vi "read serial data.vi"(8 "error in (no error)":errorcluster, 11 "serial port":refnum<visa-resource-name>) -> (0 "error out":errorcluster, 1 "readings":T2[](array[typedef]), 2 "re-synch":bool, 3 "serial port out":refnum<visa-resource-name>)   [LabVIEW 2017]
uses:
  typedefs/reading.ctl
  typedefs/readingType.ctl
  typedefs/bytes in a reading.ctl
panel:
  out "bytes at port on fail":T1=20
  out "bytes read on fail":i32
  out "Serial Settings:Number of Bytes at Serial Port":u32
  out "wrong length":bool
  out "xsum fail":bool
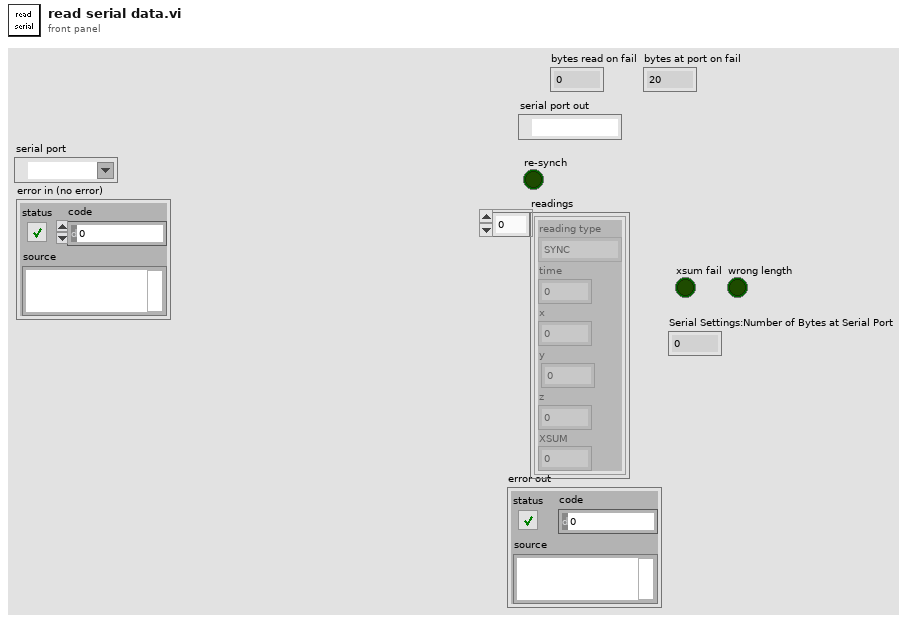
[diagram p1: front panel]
types:
  T1 = typedef "bytes in a reading.ctl" = u32
  T2 = typedef "reading.ctl" = cluster{"reading type":T3, "time":fxp<+,48,48>, "x":sgl, "y":sgl, "z":sgl, "XSUM":u8}
  T3 = typedef "readingType.ctl" = enum8{"SYNC", "DETVAL", "COILI", "MAGVEC", "ACCVEC"}
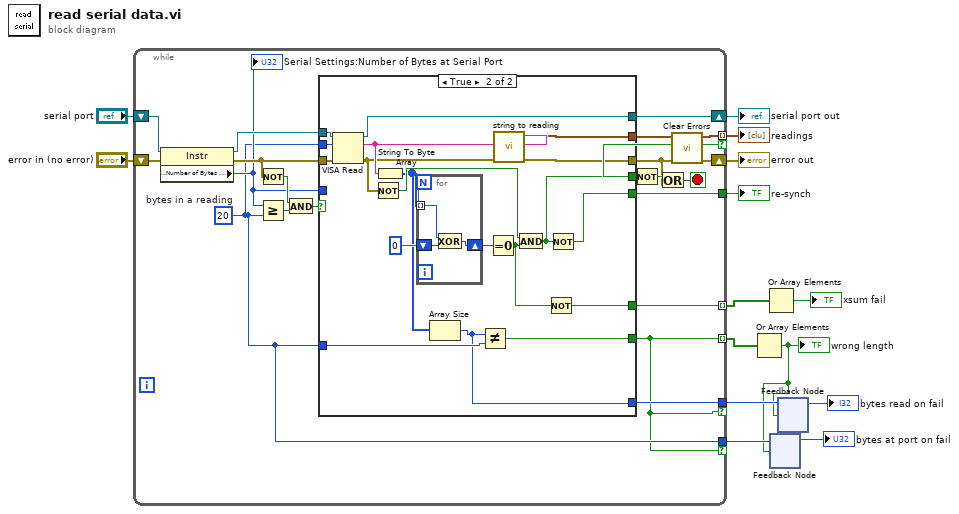
[diagram p0: block diagram]
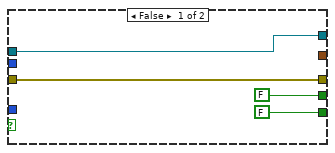
[diagram p2: hidden frame]
diagram:
  n1 = while {
    tunnel: [w27] -> w12 mode=indexing if=w23
    shift-right: [w19] -> w13
    shift-left: "error in (no error)" -> [w33]
    shift-right: [w26] -> w9
    shift-left: "serial port" -> [w25]
    tunnel: [w20] -> w10
    tunnel: [w18] -> w8 mode=indexing
    tunnel: [w15] -> w6 mode=indexing
    tunnel: [w17] -> w4 if=w15
    tunnel: [w16] -> w5 if=w15
    stop <- w21 stop-if-true
    w17 = T1 20  # bytes in a reading
    n2 = property class="Instr"(reference=w25, error in=w33) -> (reference out=w34:refnum<visa-resource-name>, error out=w30:errorcluster, "Serial Settings:Number of Bytes at Serial Port"=w28:u32)
    "Serial Settings:Number of Bytes at Serial Port" <- w28
    n3 = Not(x=w30) -> (.not. x?=w29:bool)
    n4 = Greater Or Equal?(x=w28, y=w17) -> (x >= y?=w31:bool)
    n5 = And(x=w29, y=w31) -> (x .and. y?=w32:bool)
    n6 = case shown="True" w32 {
      tunnel: w28 -> [_ _]
      tunnel: w34 -> [w36 w57]
      tunnel: w30 -> [w38 w55]
      tunnel: [w38 w49] -> w22
      tunnel: w17 -> [_ w56]
      tunnel: [FALSE w47] -> w23
      tunnel: [_ w48] -> w27
      tunnel: [FALSE w46] -> w20
      tunnel: [w36 w45] -> w26
      tunnel: w17 -> [_ w43]
      tunnel: [_ w41] -> w18
      tunnel: [_ w40] -> w15
      tunnel: [_ w39] -> w16
      frame False {
      }
      frame True {
        n7 = VISA Read(VISA resource name=w57, byte count=w56, error in (no error)=w55) -> (VISA resource name out=w45:refnum<visa-resource-name>, read buffer=w51:string, error out=w50:errorcluster)  [unwired: 1 out]
        n8 = Not(x=w50) -> (.not. x?=w52:bool)
        n9 = String To Byte Array(string=w51) -> (unsigned byte array=w44:u8[])
        n10 = for {
          tunnel: w44 -> [w60] mode=indexing
          shift-right: [w58] -> w53
          shift-left: u8 0 ("y") -> [w59]
          n11 = Exclusive Or(1:w59, 2:w60) -> (0:w58:u8)
        }
        n12 = Array Size(array=w44) -> (size(s)=w39:i32)
        n13 = Not Equal?(x=w39, y=w43) -> (x != y?=w40:bool)
        n14 = Equal To 0?(x=w53) -> (x = 0?=w42:bool)
        n15 = call "string to reading.vi"("error in (no error)"=w50, "binary string"=w51) -> ("error out"=w49:errorcluster, "reading"=w48:T2)  [unwired: 8 in]
        n16 = And(x=w52, y=w42) -> (x .and. y?=w47:bool)
        n17 = Not(x=w42) -> (.not. x?=w41:bool)
        n18 = Not(x=w47) -> (.not. x?=w46:bool)
      }
    }
    n19 = Not(x=w23) -> (.not. x?=w24:bool)
    n20 = Or(x=w24, y=w22) -> (x .or. y?=w21:bool)
    n21 = call <vilib>:"Clear Errors.vi"("error in (no error)"=w22) -> ("error out"=w19:errorcluster)  [unwired: 5 in, 1 out]
  }
  "error out" <- w13
  "readings" <- w12
  "re-synch" <- w10
  "serial port out" <- w9
  n22 = Or Array Elements(Boolean array=w6) -> (logical OR=w1:bool)
  "wrong length" <- w1
  n23 = Or Array Elements(Boolean array=w8) -> (logical OR=→"xsum fail":bool)
  n24 = feedback-in #1(w4, w1) -> ()
  n25 = feedback #1() -> (→"bytes at port on fail":T1)  [unwired: 1 in]
  n26 = feedback-in #2(w5, w1) -> ()
  n27 = feedback #2() -> (→"bytes read on fail":i32)  [unwired: 1 in]
